vi "Get Leaf Name.vi"(8 "error in (no error)":errorcluster, 11 "Leaf in":refnum<class "Leaf.lvclass">) -> (0 "error out":errorcluster, 2 "Name":string, 3 "Leaf out":refnum<class "Leaf.lvclass">)   [LabVIEW 2021, in "Bananas.lvlib" / "Leaf.lvclass"]
uses:
  Leaf.lvclass
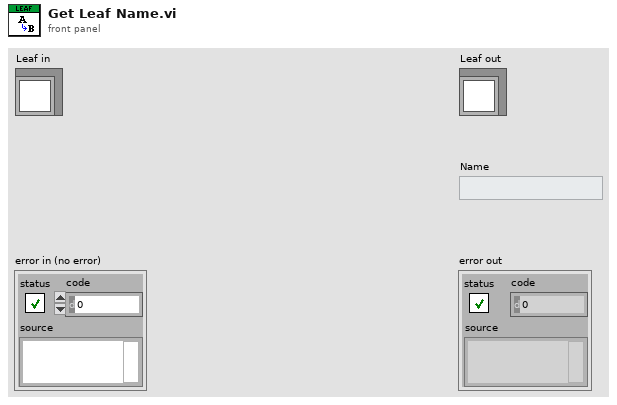
[diagram p1: front panel]
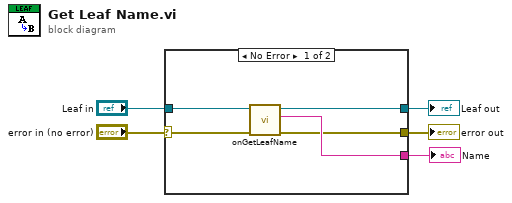
[diagram p0: block diagram]
diagram:
  n1 = case shown="No Error" "error in (no error)" {
    selector: "error in (no error)" -> [w9 w12]
    tunnel: [w6 w12] -> w4
    tunnel: [w8 w11] -> w2
    tunnel: "Leaf in" -> [w10 w11]
    tunnel: [w7 _] -> w1
    frame No Error {
      n2 = call-dynamic "onGetLeafName.vi"("error in (no error)"=w9, "Leaf in"=w10) -> ("error out"=w6:errorcluster, "Name"=w7:string, "Leaf out"=w8:refnum<class "Leaf.lvclass">)  [unwired: 7 in]
    }
    frame Error {
    }
  }
  "error out" <- w4
  "Leaf out" <- w2
  "Name" <- w1
